vi "Options Dialog.vi"(8 "error in (no error)":errorcluster, 11 "Application in":refnum<data-value>) -> (0 "error out":errorcluster, 3 "Application out":refnum<data-value>)   [LabVIEW 2015, in "Application.lvclass"]
uses:
  Application.lvclass
panel:
  in  "Plugin Folders":string
  in  "Cancel Button":bool
  in  "Save Button":bool
  in  "Project Path":path
  in  "Auto Load Project":bool
  # "Leave this field empty if project loading will handle by plugin"
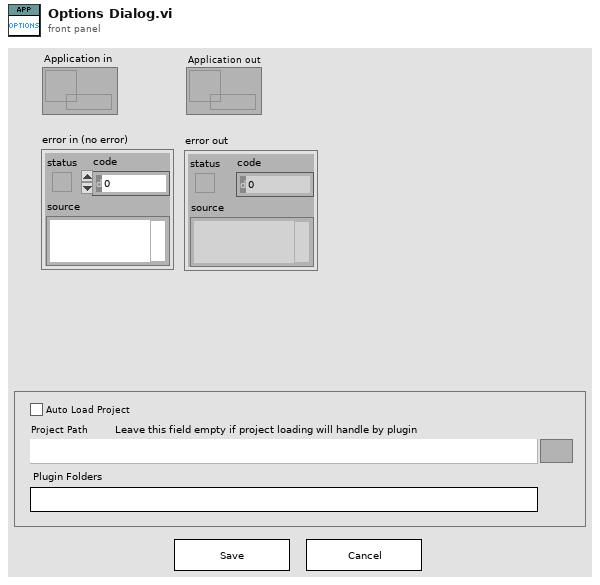
[diagram p1: front panel]
types:
  T1 = enum32{"Invalid", "Standard", "Closed", "Hidden", "Minimized", "Maximized"}
  T2 = typedef "Application Config Typedef.ctl" = cluster{"Auto Load Project":bool, "Project Path":string, "Plugin Folders":string}
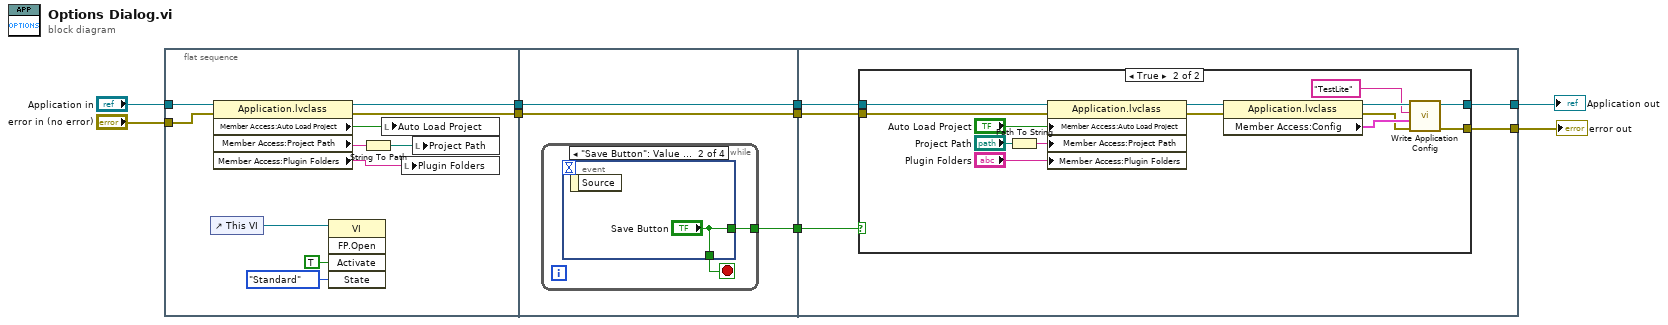
[diagram p0: block diagram]
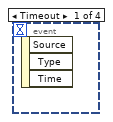
[diagram p2: hidden frame]
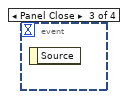
[diagram p3: hidden frame]
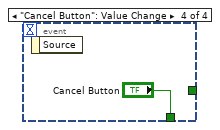
[diagram p4: hidden frame]
diagram:
  n1 = flat-sequence {
    tunnel: "Application in" -> [w19]
    tunnel: [w18] -> w9
    tunnel: "error in (no error)" -> [w14]
    tunnel: [w13] -> w2
    tunnel: w9 -> [w22]
    tunnel: [w23] -> w8
    tunnel: [w22] -> w7
    tunnel: [w21] -> w3
    tunnel: w2 -> [w21]
    tunnel: w8 -> [w28]
    tunnel: w7 -> [w32]
    tunnel: [w30] -> w5
    tunnel: w3 -> [w31]
    tunnel: [w29] -> w1
    frame #0 {
      n2 = control-ref of="This VI"() -> (w12:refnum<vi>)
      n3 = property class="Application.lvclass"(reference=w19, error in=w14) -> (reference out=w18:refnum<data-value>, error out=w13:errorcluster, "Member Access:Auto Load Project"=w17:bool, "Member Access:Project Path"=w16:string, "Member Access:Plugin Folders"=w15:string)
      n4 = invoke class="VI" method="FP.Open"(reference=w12, "Activate"=TRUE ("Activate?"), "State"=T1."Standard") -> ()  [unwired: 2 in, 5 out]
      n5 = String To Path(string=w16) -> (path=w20:path)
      n6 = local write "Auto Load Project"(w17) -> ()
      n7 = local write "Plugin Folders"(w15) -> ()
      n8 = local write "Project Path"(w20) -> ()
    }
    frame #1 {
      n9 = while {
        tunnel: [w24] -> w23
        stop <- w25 stop-if-true
        n10 = event shown="[1] \"Save Button\": Value Change" {
          selector: _ -> [_ _ _ _]
          dyn-events: _ -> [_ _ _ _]
          timeout: _ -> [_ _ _ _]
          tunnel: [_ "Save Button" _ "Cancel Button"] -> w25
          tunnel: [_ "Save Button" _ _] -> w24
          event Timeout {
            n11 = event-data() -> ()  [unwired: 1 in, 3 out]
          }
          event "Save Button": Value Change {
            n12 = event-data() -> ()  [unwired: 1 in, 1 out]
          }
          event Panel Close {
            n13 = event-data() -> ()  [unwired: 1 in, 1 out]
          }
          event "Cancel Button": Value Change {
            n14 = event-data() -> ()  [unwired: 1 in, 1 out]
          }
        }
      }
    }
    frame #2 {
      n15 = case shown="True" w28 {
        tunnel: w32 -> [w34 w47]
        tunnel: w31 -> [w33 w46]
        tunnel: [w34 w37] -> w30
        tunnel: [w33 w36] -> w29
        frame False {
        }
        frame True {
          n16 = Path To String(path="Project Path") -> (string=w44:string)
          n17 = property class="Application.lvclass"(reference=w47, error in=w46, "Member Access:Auto Load Project"="Auto Load Project", "Member Access:Project Path"=w44, "Member Access:Plugin Folders"="Plugin Folders") -> (reference out=w42:refnum<data-value>, error out=w41:errorcluster)
          n18 = property class="Application.lvclass"(reference=w42, error in=w41) -> (reference out=w38:refnum<data-value>, error out=w39:errorcluster, "Member Access:Config"=w40:T2)
          n19 = call "Write Application Config.vi"("error in (no error)"=w39, "Config Type In"=w40, "Section"="TestLite", "Application in"=w38) -> ("error out"=w36:errorcluster, "Application out"=w37:refnum<data-value>)  [unwired: 6 in]
        }
      }
    }
  }
  "error out" <- w1
  "Application out" <- w5
